vi "Setup.vi"(8 "error in (no error)":errorcluster) -> (0 "error out":errorcluster, 3 "mecanum steering frame out":refnum<class "NI_Robotics_Mecanum Steering Frame.lvclass">)   [LabVIEW 2012]
uses:
  <vilib>/robotics/Steering/Mecanum Steering Frame/NI_Robotics_Mecanum Steering Frame.lvclass
  <vilib>/robotics/Steering/Wheel/Wheel Parameters.ctl
  <vilib>/robotics/Steering/Wheel/Rotation Direction.ctl
  <vilib>/robotics/Steering/Mecanum Wheel/Create Mecanum Wheel.vi
  <vilib>/robotics/Steering/Mecanum Steering Frame/Create Mecanum Steering Frame.vi
  <vilib>/robotics/Steering/Wheel/NI_Robotics_Wheel.lvclass
  <vilib>/robotics/Steering/Mecanum Wheel/NI_Robotics_Mecanum Wheel.lvclass
  <vilib>/robotics/Steering/Steering Frame/NI_Robotics_Steering Frame.lvclass
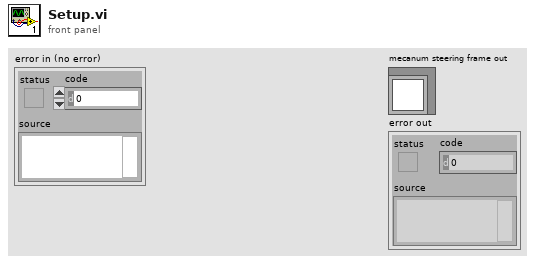
[diagram p1: front panel]
types:
  T1 = typedef "NI_Robotics_Wheel.lvclass/Wheel Parameters.ctl" = cluster{"wheel radius":dbl, "gear ratio":dbl, "forward rotation direction":T2}
  T2 = typedef "NI_Robotics_Wheel.lvclass/Rotation Direction.ctl" = u16
  T3 = cluster{"mecanum wheel out":refnum<class "NI_Robotics_Mecanum Wheel.lvclass">, "mecanum wheel out":refnum<class "NI_Robotics_Mecanum Wheel.lvclass">, "mecanum wheel out":refnum<class "NI_Robotics_Mecanum Wheel.lvclass">, "mecanum wheel out":refnum<class "NI_Robotics_Mecanum Wheel.lvclass">}
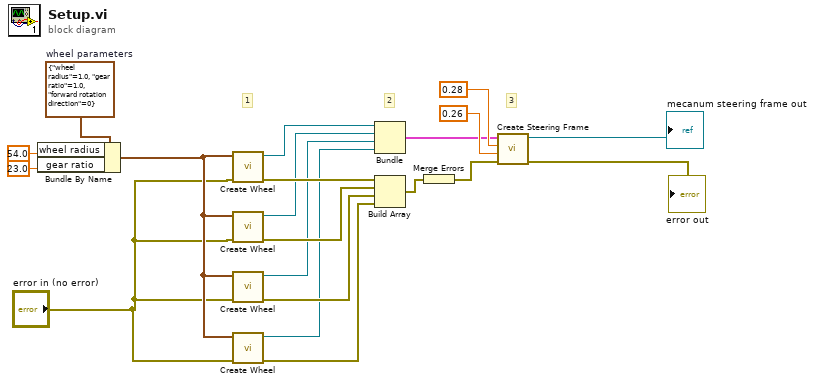
[diagram p0: block diagram]
diagram:
  w5 = T1 {"wheel radius"=1.0, "gear ratio"=1.0, "forward rotation direction"=0}  # wheel parameters
  # "3"
  # "2"
  # "1"
  n1 = Bundle By Name(cluster=w5, "wheel radius"=54.0, "gear ratio"=23.0) -> (w4:T1)
  n2 = call-poly <vilib>:"Create Wheel.vi"("error in (no error)"="error in (no error)", "wheel parameters"=w4) -> ("error out"=w15:errorcluster, "mecanum wheel out"=w8:refnum<class "NI_Robotics_Mecanum Wheel.lvclass">)  [unwired: 8 in]
  n3 = call-poly <vilib>:"Create Wheel.vi"("error in (no error)"="error in (no error)", "wheel parameters"=w4) -> ("error out"=w16:errorcluster, "mecanum wheel out"=w9:refnum<class "NI_Robotics_Mecanum Wheel.lvclass">)  [unwired: 8 in]
  n4 = call-poly <vilib>:"Create Wheel.vi"("error in (no error)"="error in (no error)", "wheel parameters"=w4) -> ("error out"=w17:errorcluster, "mecanum wheel out"=w10:refnum<class "NI_Robotics_Mecanum Wheel.lvclass">)  [unwired: 8 in]
  n5 = call-poly <vilib>:"Create Wheel.vi"("error in (no error)"="error in (no error)", "wheel parameters"=w4) -> ("error out"=w19:errorcluster, "mecanum wheel out"=w11:refnum<class "NI_Robotics_Mecanum Wheel.lvclass">)  [unwired: 8 in]
  n6 = Bundle("mecanum wheel out"=w8, "mecanum wheel out"=w9, "mecanum wheel out"=w10, "mecanum wheel out"=w11) -> (w12:T3)  [unwired: 1 in]
  n7 = Build Array(w15, w16, w17, w19) -> (w18:errorcluster[])
  n8 = Merge Errors(w18) -> (w20:errorcluster)
  n9 = call-poly <vilib>:"Create Steering Frame.vi"("error in (no error)"=w20, "wheel separation length"=0.26, "wheel separation width"=0.28, "wheels"=w12) -> ("error out"=→"error out":errorcluster, "mecanum steering frame out"=→"mecanum steering frame out":refnum<class "NI_Robotics_Mecanum Steering Frame.lvclass">)  [unwired: 6 in]
